vi "LoadSlide.vi"(2 "slide background":u32(colorbox), 3 "Slide path":path, 4 "object in":refnum<vi>) -> (0 "Slide path":path, 1 "object out":refnum<vi>)   [LabVIEW 2010]
uses:
  LVPresent_Globals.vi
  <vilib>/picture/3D Picture Control/NI_3D Picture Control.lvlib
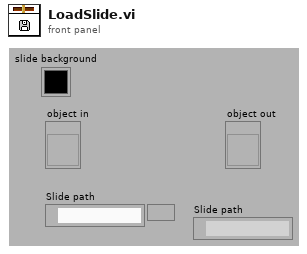
[diagram p1: front panel]
types:
  T1 = enum16{"As a Decal", "With Modulation", "With Blending", "As a replacement"}
  T2 = typedef "LVBoundsTypeDef.ctl" = cluster{"Width":u32, "Height":u32}
  T3 = typedef "imagedata.ctl" = cluster{"image type":i32, "image depth":i32, "image":u8[], "mask":u8[], "colors":u32[], "Rectangle":cluster{"left":i16, "top":i16, "right":i16, "bottom":i16}}
  T4 = cluster{"Resolution":i32, "Resolution":i32, "Width":u32, "Height":u32}
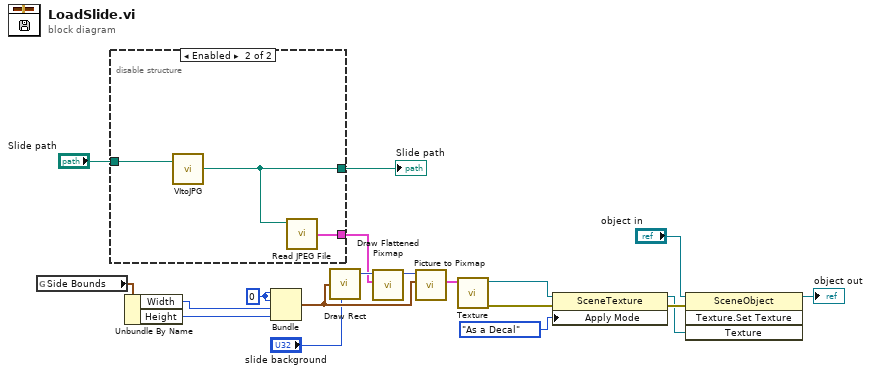
[diagram p0: block diagram]
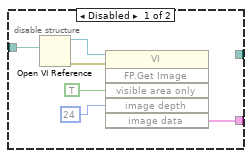
[diagram p2: hidden frame]
diagram:
  w16 = 0 ("Resolution")
  n1 = global read "LVPresent_Globals.vi" "Side Bounds"() -> (w2:T2)
  n2 = disable-structure shown="Enabled" {
    disable-tunnel: [w25 w27] -> w1
    disable-tunnel: [_ w26] -> w14
    disable-tunnel: "Slide path" -> [w20 w28]
    frame Disabled {
      n3 = Open VI Reference(vi path=w20) -> (vi reference=w21:refnum<vi>, error out=w22:errorcluster)  [unwired: 5 in]
      n4 = invoke class="VI" method="FP.Get Image"(reference=w21, error in=w22, "visible area only"=TRUE ("Visible Area Only"), "image depth"=24 ("Image Depth")) -> ("image data"=w25:T3)  [unwired: 2 in, 5 out]
    }
    frame Enabled {
      n5 = call "VItoJPG.vi"("Dest"=w28) -> ("appended path"=w26:path)  [unwired: 1 in]
      n6 = call <vilib>:"Read JPEG File.vi"("path to JPEG file"=w26) -> ("image data"=w27:T3)  [unwired: 8 in, 2 out]
    }
  }
  "Slide path" <- w14
  n7 = Unbundle By Name(w2) -> ("Width"=w5:u32, "Height"=w4:u32)
  n8 = Bundle("Resolution"=w16, "Resolution"=w16, "Width"=w5, "Height"=w4) -> (w18:T4)  [unwired: 1 in]
  n9 = call <vilib>:"Draw Rect.vi"("rect"=w18, "color(black)"="slide background") -> ("new picture"=w15:picture)  [unwired: 7 in]
  n10 = call <vilib>:"Draw Flattened Pixmap.vi"("image data"=w1, "picture"=w15) -> ("new picture"=w17:picture)  [unwired: 7 in]
  n11 = call <vilib>:"Picture to Pixmap.vi"("rect"=w18, "picture"=w17) -> ("image data"=w19:T3)  [unwired: 8 in, 1 out]
  n12 = call <vilib>:"Texture.vi"("Image"=w19) -> ("error out"=w9:errorcluster, "New Texture Refnum"=w7:refnum<vi>)  [unwired: 1 in, 8 out]
  n13 = property class="SceneTexture"(reference=w7, error in=w9, "Apply Mode"=T1."As a Decal") -> (reference out=w8:refnum<vi>, error out=w10:errorcluster)
  n14 = invoke class="SceneObject" method="Texture.Set Texture"(reference="object in", error in=w10, "Texture"=w8) -> (reference out=→"object out":refnum<vi>)  [unwired: 1 in, 3 out]
